vi "BRig_dataLC_ENL_First_Delay_l2.vi"() -> (2 "output_ENL_First_Delay_l2":i32)   [LabVIEW 2014]
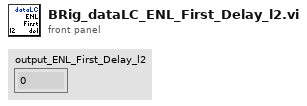
[diagram p1: front panel]
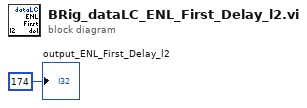
[diagram p0: block diagram]
diagram:
  "output_ENL_First_Delay_l2" <- 174 ("output_iBlock")
